vi "ship movement.vi"(4 "key input":T1(ring), 6 "orientation":i32, 7 "current position drawing":u32[][](array[numeric]), 9 "column":i32, 10 "row":i32, 11 "all  position drawings":T2) -> (1 "next orientation":i32, 2 "next column":i32, 3 "next row":i32, 5 "next position drawing":u32[][](array[numeric]))   [LabVIEW 2019]
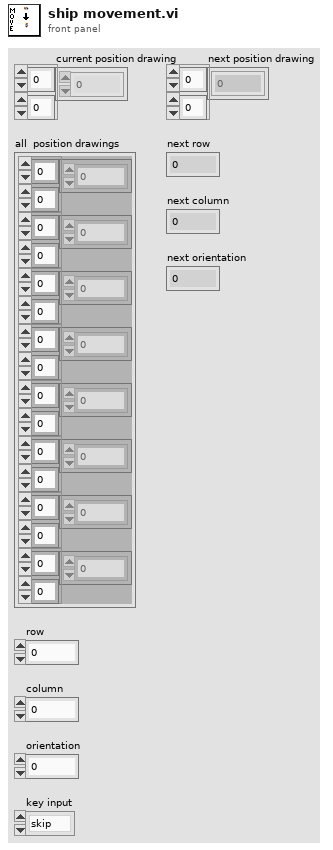
[diagram p1: front panel]
types:
  T1 = enum16{"skip", "prawo", "lewo", "ruch", "strzal"}
  T2 = cluster{u32[][], u32[][], u32[][], u32[][], u32[][], u32[][], u32[][], u32[][]}
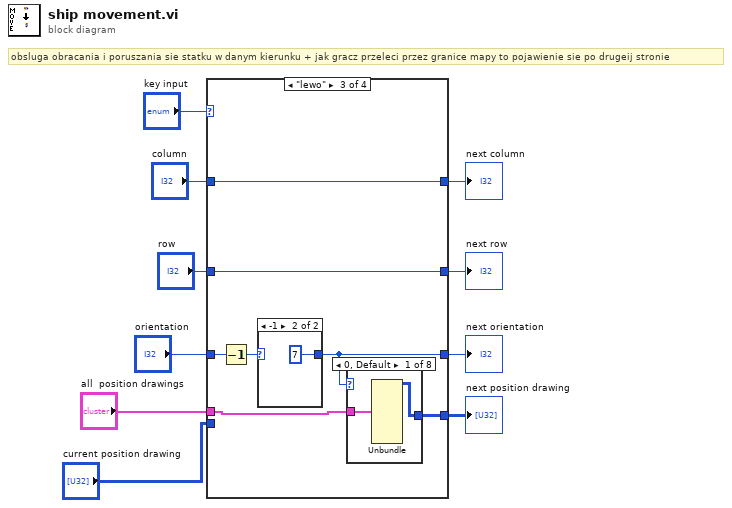
[diagram p0: block diagram]
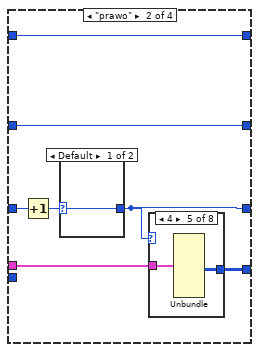
[diagram p3: hidden frame]
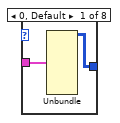
[diagram p4: hidden frame]
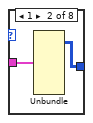
[diagram p5: hidden frame]
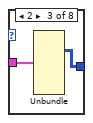
[diagram p6: hidden frame]
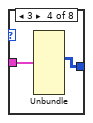
[diagram p7: hidden frame]
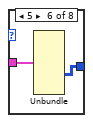
[diagram p8: hidden frame]
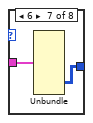
[diagram p9: hidden frame]
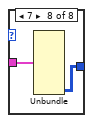
[diagram p10: hidden frame]
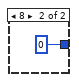
[diagram p11: hidden frame]
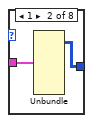
[diagram p12: hidden frame]
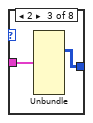
[diagram p13: hidden frame]
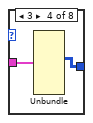
[diagram p14: hidden frame]
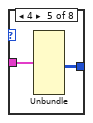
[diagram p15: hidden frame]
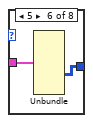
[diagram p16: hidden frame]
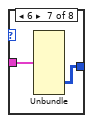
[diagram p17: hidden frame]
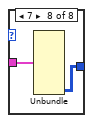
[diagram p18: hidden frame]
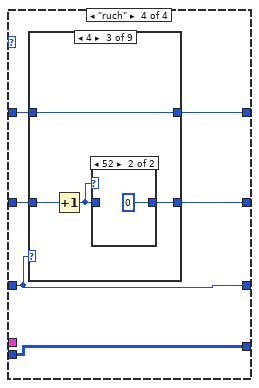
[diagram p20: hidden frame]
diagram:
  # "obsluga obracania i poruszania sie statku w danym kierunku + jak gracz przeleci przez granice mapy to pojawienie sie po drugeij stronie"
  n1 = case shown="\"lewo\"" "key input" {
    tunnel: "row" -> [w14 w20 w46 w65]
    tunnel: [w14 w20 w46 w67] -> w3
    tunnel: "column" -> [w13 w21 w45 w66]
    tunnel: [w13 w21 w45 w68] -> w5
    tunnel: "all  position drawings" -> [_ w16 w43 _]
    tunnel: [w12 w15 w42 w70] -> w7
    tunnel: "current position drawing" -> [w12 _ _ w70]
    tunnel: "orientation" -> [w11 w19 w40 w69]
    tunnel: [w11 w17 w41 w69] -> w10
    frame "skip", Default {
    }
    frame "prawo" {
      n2 = Increment(x=w19) -> (x+1=w18:i32)
      n3 = case shown="Default" w18 {
        selector: w18 -> [w38 _]
        tunnel: [w38 0] -> w17
        frame Default {
        }
        frame 8 {
        }
      }
      n4 = case shown="4" w17 {
        tunnel: w16 -> [w23 w25 w27 w29 w31 w33 w35 w37]
        tunnel: [w22 w24 w26 w28 w30 w32 w34 w36] -> w15
        frame 0, Default {
          n5 = Unbundle(w23) -> (w22:u32[][])  [unwired: 7 out]
        }
        frame 1 {
          n6 = Unbundle(w25) -> (w24:u32[][])  [unwired: 7 out]
        }
        frame 2 {
          n7 = Unbundle(w27) -> (w26:u32[][])  [unwired: 7 out]
        }
        frame 3 {
          n8 = Unbundle(w29) -> (w28:u32[][])  [unwired: 7 out]
        }
        frame 4 {
          n9 = Unbundle(w31) -> (w30:u32[][])  [unwired: 7 out]
        }
        frame 5 {
          n10 = Unbundle(w33) -> (w32:u32[][])  [unwired: 7 out]
        }
        frame 6 {
          n11 = Unbundle(w35) -> (w34:u32[][])  [unwired: 7 out]
        }
        frame 7 {
          n12 = Unbundle(w37) -> (w36:u32[][])  [unwired: 7 out]
        }
      }
    }
    frame "lewo" {
      n13 = Decrement(x=w40) -> (x-1=w44:i32)
      n14 = case shown="-1" w44 {
        selector: w44 -> [w63 _]
        tunnel: [w63 7] -> w41
        frame Default {
        }
        frame -1 {
        }
      }
      n15 = case shown="0, Default" w41 {
        tunnel: w43 -> [w48 w50 w52 w54 w56 w58 w60 w62]
        tunnel: [w47 w49 w51 w53 w55 w57 w59 w61] -> w42
        frame 0, Default {
          n16 = Unbundle(w48) -> (w47:u32[][])  [unwired: 7 out]
        }
        frame 1 {
          n17 = Unbundle(w50) -> (w49:u32[][])  [unwired: 7 out]
        }
        frame 2 {
          n18 = Unbundle(w52) -> (w51:u32[][])  [unwired: 7 out]
        }
        frame 3 {
          n19 = Unbundle(w54) -> (w53:u32[][])  [unwired: 7 out]
        }
        frame 4 {
          n20 = Unbundle(w56) -> (w55:u32[][])  [unwired: 7 out]
        }
        frame 5 {
          n21 = Unbundle(w58) -> (w57:u32[][])  [unwired: 7 out]
        }
        frame 6 {
          n22 = Unbundle(w60) -> (w59:u32[][])  [unwired: 7 out]
        }
        frame 7 {
          n23 = Unbundle(w62) -> (w61:u32[][])  [unwired: 7 out]
        }
      }
    }
    frame "ruch" {
      n24 = case shown="4" w69 {
        tunnel: [w74 w80 w90 w93 w104 w113 w119 w121 w132] -> w68
        tunnel: [w72 w78 w88 w96 w106 w110 w120 w124 w134] -> w67
        tunnel: w66 -> [w74 w81 w90 w94 w105 w112 w119 w122 w133]
        tunnel: w65 -> [w73 w77 w89 w97 w106 w109 w120 w125 w134]
        frame 0 {
          n25 = Decrement(x=w73) -> (x-1=w71:i32)
          n26 = case shown="-1" w71 {
            tunnel: [w75 51] -> w72
            tunnel: w71 -> [w75 _]
            frame Default {
            }
            frame -1 {
            }
          }
        }
        frame 3 {
          n27 = Increment(x=w81) -> (x+1=w82:i32)
          n28 = Increment(x=w77) -> (x+1=w79:i32)
          n29 = case shown="55" w82 {
            tunnel: [w85 0] -> w80
            tunnel: w82 -> [w85 _]
            frame Default {
            }
            frame 55 {
            }
          }
          n30 = case shown="52" w79 {
            tunnel: [w83 0] -> w78
            tunnel: w79 -> [w83 _]
            frame Default {
            }
            frame 52 {
            }
          }
        }
        frame 4 {
          n31 = Increment(x=w89) -> (x+1=w87:i32)
          n32 = case shown="52" w87 {
            tunnel: [w91 0] -> w88
            tunnel: w87 -> [w91 _]
            frame Default {
            }
            frame 52 {
            }
          }
        }
        frame 5 {
          n33 = Decrement(x=w94) -> (x-1=w95:i32)
          n34 = Increment(x=w97) -> (x+1=w98:i32)
          n35 = case shown="-1" w95 {
            tunnel: [w99 54] -> w93
            tunnel: w95 -> [w99 _]
            frame Default {
            }
            frame -1 {
            }
          }
          n36 = case shown="52" w98 {
            tunnel: [w101 0] -> w96
            tunnel: w98 -> [w101 _]
            frame Default {
            }
            frame 52 {
            }
          }
        }
        frame 6 {
          n37 = Decrement(x=w105) -> (x-1=w103:i32)
          n38 = case shown="-1" w103 {
            tunnel: [w107 54] -> w104
            tunnel: w103 -> [w107 _]
            frame Default {
            }
            frame -1 {
            }
          }
        }
        frame 7 {
          n39 = Decrement(x=w112) -> (x-1=w114:i32)
          n40 = Decrement(x=w109) -> (x-1=w111:i32)
          n41 = case shown="-1" w114 {
            tunnel: [w117 54] -> w113
            tunnel: w114 -> [w117 _]
            frame Default {
            }
            frame -1 {
            }
          }
          n42 = case shown="-1" w111 {
            tunnel: [w115 51] -> w110
            tunnel: w111 -> [w115 _]
            frame Default {
            }
            frame -1 {
            }
          }
        }
        frame Default {
        }
        frame 1 {
          n43 = Increment(x=w122) -> (x+1=w123:i32)
          n44 = Decrement(x=w125) -> (x-1=w126:i32)
          n45 = case shown="55" w123 {
            tunnel: [w127 0] -> w121
            tunnel: w123 -> [w127 _]
            frame Default {
            }
            frame 55 {
            }
          }
          n46 = case shown="-1" w126 {
            tunnel: [w129 51] -> w124
            tunnel: w126 -> [w129 _]
            frame Default {
            }
            frame -1 {
            }
          }
        }
        frame 2 {
          n47 = Increment(x=w133) -> (x+1=w131:i32)
          n48 = case shown="55" w131 {
            tunnel: [w135 0] -> w132
            tunnel: w131 -> [w135 _]
            frame Default {
            }
            frame 55 {
            }
          }
        }
      }
    }
  }
  "next orientation" <- w10
  "next position drawing" <- w7
  "next column" <- w5
  "next row" <- w3
